vi "calibrateEvent.vi"(8 "error in (no error)":errorcluster, 11 "ScriptEvent in":refnum<class "ScriptEvent.lvclass">) -> (0 "error out":errorcluster, 3 "ScriptEvent out":refnum<class "ScriptEvent.lvclass">)   [LabVIEW 2011, in "Tools.lvlib" / "Scripting.lvlib" / "ScriptEvent.lvclass"]
uses:
  ScriptEvent.lvclass
  ScriptEvent.lvclass/ScriptEvent.ctl
  DatabaseHelpers/Database Objects/Channel/Channel.lvclass
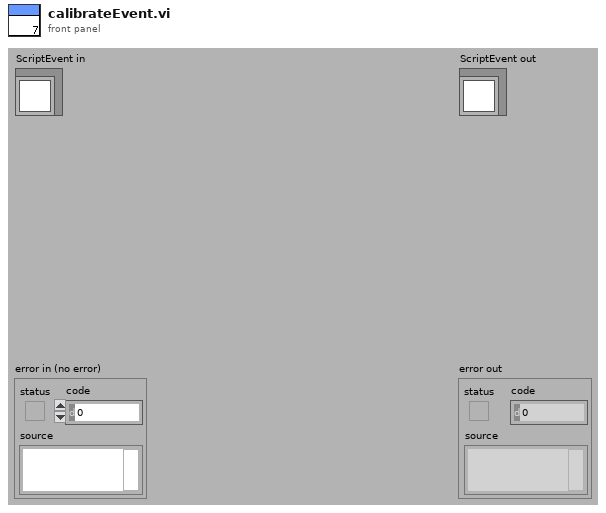
[diagram p1: front panel]
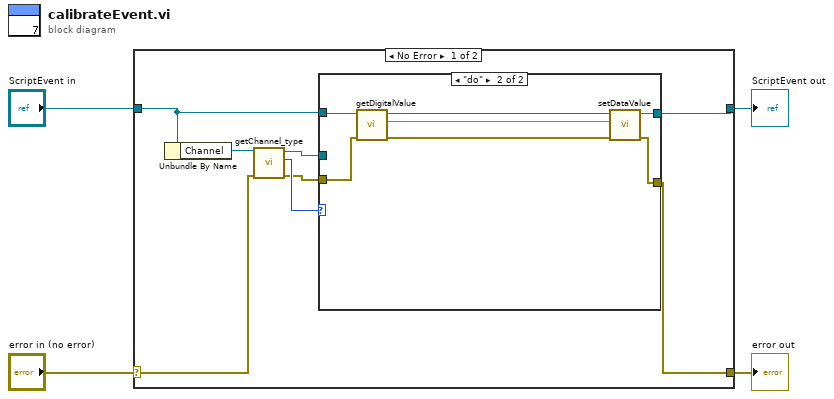
[diagram p0: block diagram]
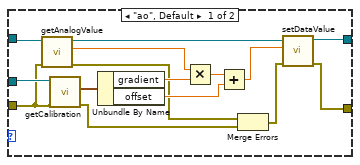
[diagram p2: hidden frame]
diagram:
  n1 = case shown="No Error" "error in (no error)" {
    selector: "error in (no error)" -> [w10 w36]
    tunnel: [w6 w36] -> w3
    tunnel: [w5 w35] -> w1
    tunnel: "ScriptEvent in" -> [w7 w35]
    frame No Error {
      n2 = Unbundle By Name(w7) -> ("Channel"=w12:refnum<class "Channel.lvclass">)
      n3 = call "getChannel_type.vi"("error in (no error)"=w10, "Channel.lvclass in"=w12) -> ("error out"=w9:errorcluster, "channel_type"=w11:enum16{"ao", "do", "ai", "di", "rf"}, "Channel.lvclass out"=w8:refnum<class "Channel.lvclass">)  [unwired: 7 in]
      n4 = case shown="\"do\"" w11 {
        tunnel: w9 -> [w25 w32]
        tunnel: w8 -> [w26 _]
        tunnel: w7 -> [w27 w33]
        tunnel: [w14 w28] -> w6
        tunnel: [w13 w34] -> w5
        frame "ao", Default {
          n5 = call "getAnalogValue.vi"("error in (no error)"=w25, "ScriptEvent in"=w27) -> ("error out"=w17:errorcluster, "analogValue"=w23:dbl, "ScriptEvent out"=w20:refnum<class "ScriptEvent.lvclass">)  [unwired: 7 in]
          n6 = call "getCalibration.vi"("error in (no error)"=w25, "Channel.lvclass in"=w26) -> ("error out"=w16:errorcluster, "calibration"=w24:cluster{"gradient":dbl, "offset":dbl})  [unwired: 7 in, 1 out]
          n7 = Unbundle By Name(w24) -> ("gradient"=w22:dbl, "offset"=w19:dbl)
          n8 = Multiply(x=w23, y=w22) -> (x*y=w21:dbl)
          n9 = Add(x=w21, y=w19) -> (x+y=w18:dbl)
          n10 = Merge Errors(w17, w16) -> (w15:errorcluster)
          n11 = call "setDataValue.vi"("error in (no error)"=w15, "dataValue"=w18, "ScriptEvent.lvclass in"=w20) -> ("error out"=w14:errorcluster, "ScriptEvent.lvclass out"=w13:refnum<class "ScriptEvent.lvclass">)  [unwired: 7 in]
        }
        frame "do" {
          n12 = call "getDigitalValue.vi"("error in (no error)"=w32, "ScriptEvent in"=w33) -> ("error out"=w31:errorcluster, "digitalValue"=w29:dbl, "ScriptEvent out"=w30:refnum<class "ScriptEvent.lvclass">)  [unwired: 7 in]
          n13 = call "setDataValue.vi"("error in (no error)"=w31, "dataValue"=w29, "ScriptEvent.lvclass in"=w30) -> ("error out"=w28:errorcluster, "ScriptEvent.lvclass out"=w34:refnum<class "ScriptEvent.lvclass">)  [unwired: 7 in]
        }
      }
    }
    frame Error {
    }
  }
  "error out" <- w3
  "ScriptEvent out" <- w1
